vi "TestStand_Control ( Exit_Callback ).vi"(4 "TestStand UI Data":T1, 6 "Control Ref":refnum<k7>, 7 "Event Common Data":T2) -> ()   [LabVIEW 2018, in "TestStand_Control.lvlib"]
uses:
  Module_Controls/TestStand UI Data.ctl
  TestStand_Control.lvlib
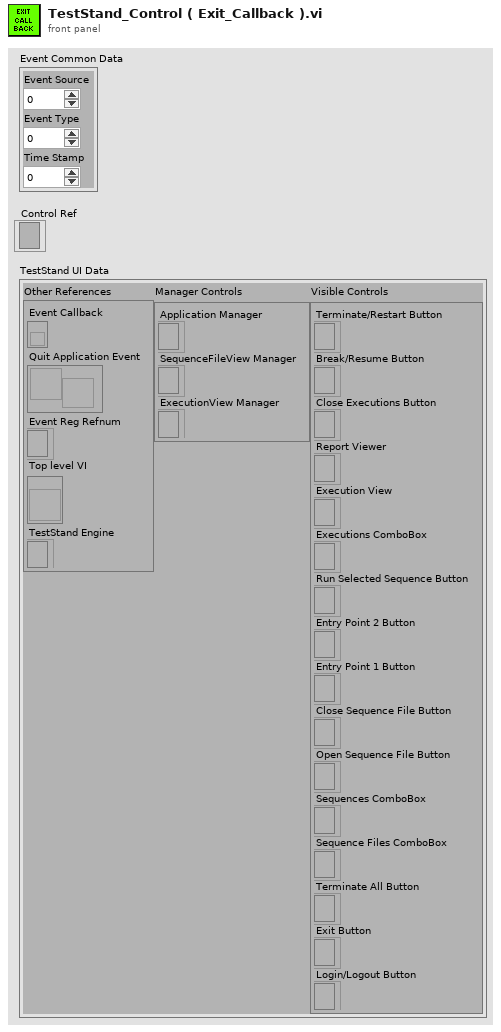
[diagram p1: front panel]
types:
  T1 = typedef "TestStand_Control.lvlib/TestStand UI Data.ctl" = cluster{"Other References":cluster{"Event Callback":refnum<k27>, "Quit Application Event":refnum<user-event>, "Event Reg Refnum":refnum<event-registration>, "Top level VI":refnum<vi>, "TestStand Engine":refnum<k7>}, "Manager Controls":cluster{"Application Manager":refnum<k7>, "SequenceFileView Manager":refnum<k7>, "ExecutionView Manager":refnum<k7>}, "Visible Controls":cluster{"Terminate/Restart Button":refnum<k7>, "Break/Resume Button":refnum<k7>, "Close Executions Button":refnum<k7>, "Report Viewer":refnum<k7>, "Execution View":refnum<k7>, "Executions ComboBox":refnum<k7>, "Run Selected Sequence Button":refnum<k7>, "Entry Point 2 Button":refnum<k7>, "Entry Point 1 Button":refnum<k7>, "Close Sequence File Button":refnum<k7>, "Open Sequence File Button":refnum<k7>, "Sequences ComboBox":refnum<k7>, "Sequence Files ComboBox":refnum<k7>, "Terminate All Button":refnum<k7>, "Exit Button":refnum<k7>, "Login/Logout Button":refnum<k7>}}
  T2 = cluster{"Event Source":i32, "Event Type":u32, "Time Stamp":u32}
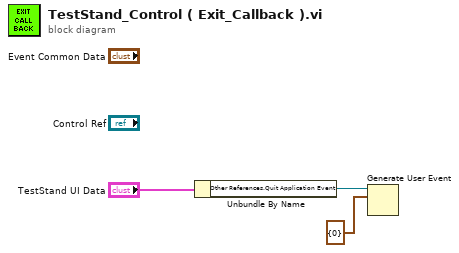
[diagram p0: block diagram]
diagram:
  n1 = Unbundle By Name("TestStand UI Data") -> ("Other References.Quit Application Event"=w2:refnum<user-event>)
  n2 = Generate User Event(user event=w2, event data cluster=cluster{"Number":i32} {"Number"=0} ("event data")) -> ()  [unwired: 2 in, 2 out]
